vi "Calculate Histogram from Pairs.vi"(5 "Slave Histogram":bool, 7 "Switch X/Y":bool, 11 "Matched Values":T1(array[cluster])) -> (3 "Histogram Data":cluster{cluster{dbl, dbl}[]}[](array[cluster]))   [LabVIEW 2019, in "Muon Data Post-Processing.lvlib"]
uses:
  Muon Data Post-Processing.lvlib
  <vilib>/Utility/miscctls.llb/LVMapReplaceAction.ctl
  <vilib>/Analysis/1siggen.llb/Ramp Pattern by Delta.vi
  <vilib>/Analysis/NI_AALBase.lvlib
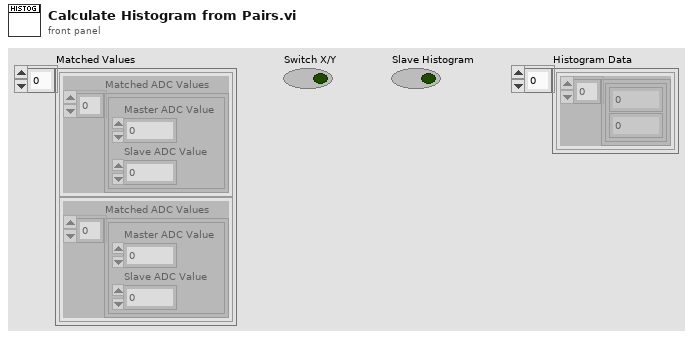
[diagram p1: front panel]
types:
  T1 = cluster{"Matched ADC Values":cluster{"Master ADC Value":i32, "Slave ADC Value":i32}[]}[]
  T2 = typedef "LVMapReplaceAction.ctl" = enum32{"Modify Entry only if found", "Add or Modify Entry", "Delete Entry"}
  T3 = cluster{"Master ADC Value":i32, "Slave ADC Value":i32}[]
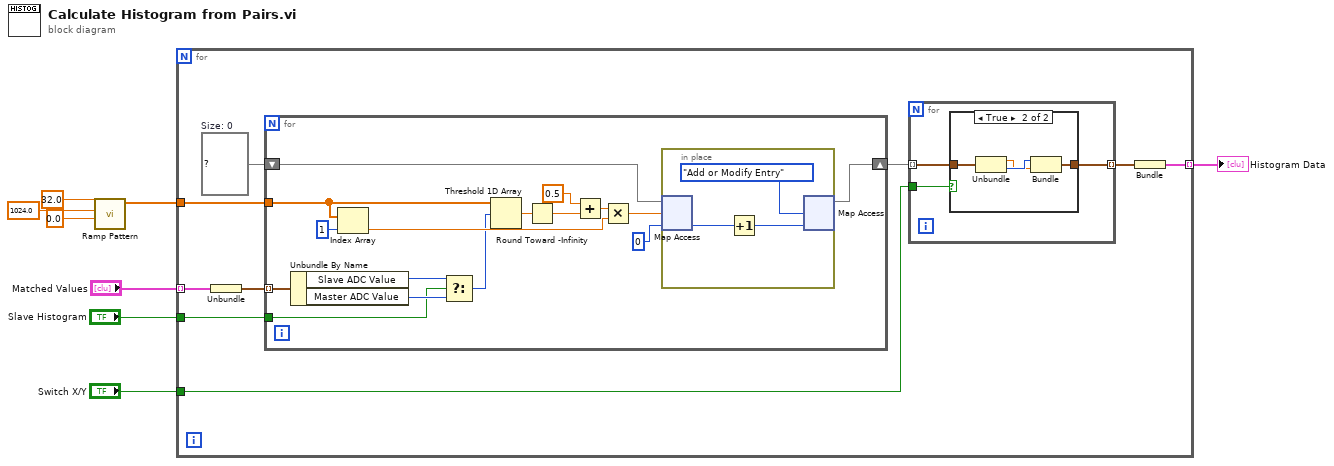
[diagram p0: block diagram]
diagram:
  n1 = call-poly <vilib>:"Ramp Pattern.vi"("start"=0.0, "end"=1024.0, "delta"=32.0) -> ("Ramp Pattern"=w5:dbl[])  [unwired: 6 in, 2 out]
  n2 = for {
    tunnel: w5 -> [w17]
    tunnel: [w10] -> w4 mode=indexing
    tunnel: "Switch X/Y" -> [w14]
    tunnel: "Slave Histogram" -> [w13]
    tunnel: "Matched Values" -> [w11] mode=indexing
    w16 = map{dbl, i32} {}  # Size: 0
    n3 = Unbundle(w11) -> ("Matched ADC Values"=w12:T3)
    n4 = for {
      tunnel: w12 -> [w41] mode=indexing
      shift-right: [w32] -> w15
      shift-left: w16 -> [w31]
      tunnel: w17 -> [w30]
      tunnel: w13 -> [w26]
      n5 = Unbundle By Name(w41) -> ("Slave ADC Value"=w29:i32, "Master ADC Value"=w28:i32)
      n6 = Index Array(array=w30, index=1) -> (element=w40:dbl)
      n7 = Select(t=w29, s=w26, f=w28) -> (s? t:f=w27:i32)
      n8 = Threshold 1D Array(2:w27, 3:w30) -> (0:w39:dbl)  [unwired: 1 in]
      n9 = Round Toward -Infinity(1:w39) -> (0:w38:dbl)
      n10 = Add(x=0.5, y=w38) -> (x+y=w37:dbl)
      n11 = Multiply(x=w37, y=w40) -> (x*y=w34:dbl)
      n12 = in-place {
        n13 = in-place-map #1(w31, w34, 0) -> (w44:i32)  [unwired: 1 out]
        n14 = Increment(x=w44) -> (x+1=w43:i32)
        n15 = in-place-map #1(w43, LVMapReplaceAction."Add or Modify Entry" ("action")) -> (w32:map{dbl, i32})  [unwired: 2 out]
      }
    }
    n16 = for {
      tunnel: w15 -> [w19] mode=indexing
      tunnel: [w20] -> w9 mode=indexing
      tunnel: w14 -> [w18]
      n17 = case shown="True" w18 {
        tunnel: [w21 w22] -> w20
        tunnel: w19 -> [w21 w25]
        frame False {
        }
        frame True {
          n18 = Unbundle(w25) -> (w23:dbl, w24:i32)
          n19 = Bundle(w24, w23) -> (w22:cluster{i32, dbl})  [unwired: 1 in]
        }
      }
    }
    n20 = Bundle(w9) -> (w10:cluster{cluster{dbl, dbl}[]})  [unwired: 1 in]
  }
  "Histogram Data" <- w4
